vi "Get Self Queue.vi"(8 "error in (no error)":errorcluster, 11 "Actor API in":refnum<class "Actor API.lvclass">) -> (0 "error out":errorcluster, 2 "Self Queue":refnum<class "Priority Message Queue.lvclass">, 3 "Actor API out":refnum<class "Actor API.lvclass">)   [LabVIEW 2020, in "Artifex.lvlib" / "Actor API.lvclass"]
uses:
  Actor API.lvclass
  Priority Message Queue/Priority Message Queue.lvclass
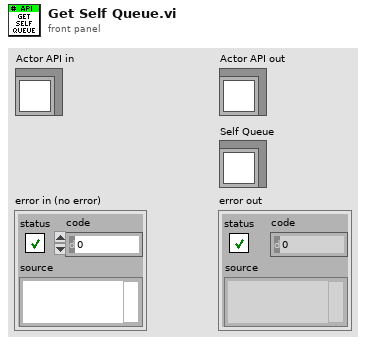
[diagram p1: front panel]
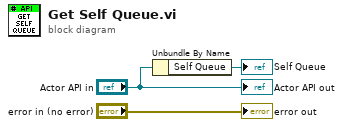
[diagram p0: block diagram]
diagram:
  n1 = Unbundle By Name("Actor API in") -> ("Self Queue"=→"Self Queue":refnum<class "Priority Message Queue.lvclass">)
  "error out" <- "error in (no error)"
  "Actor API out" <- "Actor API in"
